vi "5668 Initialize Scan with External LO.vi"(8 "error in (no error)":errorcluster, 10 "Start Carrier Frequency (Hz)":dbl=4000000000.0 format="%#_13p", 11 "Instrument Handles in":T1={"Resource Name RFSA"="RFSA", "Resource Name RFSG LO Generation"="RFSG"}) -> (0 "error out":errorcluster, 3 "Instrument Handles out":T1={"Resource Name RFSA"="RFSA", "Resource Name RFSG LO Generation"="RFSG"})   [LabVIEW 2017]
uses:
  Instrument Handles.ctl
  <instrlib>/niRFSA/niRFSA.llb/niRFSA Acquisition Types.ctl
  <instrlib>/niRFSA/niRFSA.llb/niRFSA Ref Clock Sources.ctl
panel:
  in  "resource name":refnum<k15>="PXI1Slot17"
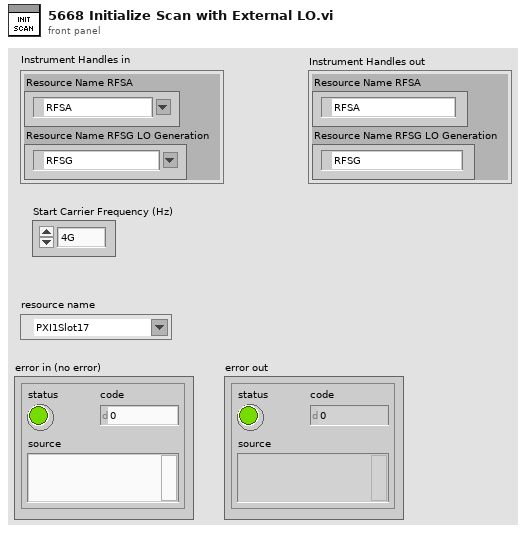
[diagram p1: front panel]
types:
  T1 = typedef "Instrument Handles.ctl" = cluster{"Resource Name RFSA":refnum<k15>, "Resource Name RFSG LO Generation":refnum<k15>}
  T2 = typedef "niRFSA Ref Clock Sources.ctl" = string
  T3 = typedef "niRFSA Acquisition Types.ctl" = i32
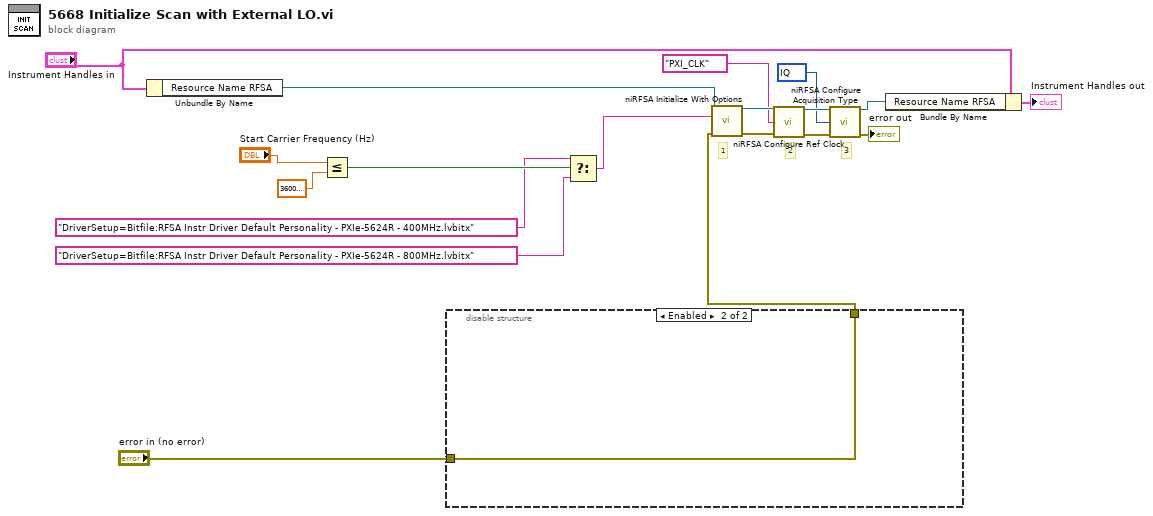
[diagram p0: block diagram]
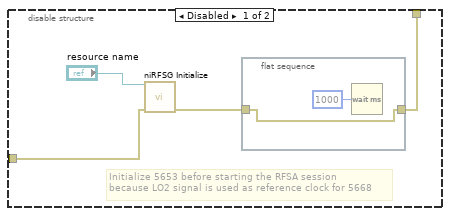
[diagram p2: hidden frame]
diagram:
  w14 = T3 100 items=["IQ"=100, "Spectrum"=101] ("acquisition type")
  # "3"
  # "2"
  # "1"
  n1 = Unbundle By Name("Instrument Handles in") -> ("Resource Name RFSA"=w12:refnum<k15>)
  n2 = Less Or Equal?(x="Start Carrier Frequency (Hz)", y=3600000000.0) -> (x <= y?=w10:bool)
  n3 = disable-structure shown="Enabled" {
    disable-tunnel: "error in (no error)" -> [w22 w26]
    disable-tunnel: [w20 w26] -> w1
    frame Disabled {
      # "Initialize 5653 before starting the RFSA session\nbecause LO2 signal is used as reference clock for 5668"
      n4 = call <instrlib>:"niRFSG Initialize.vi"("resource name"="resource name", "error in"=w22) -> ("error out"=w21:errorcluster)  [unwired: 12 in, 1 out]
      n5 = flat-sequence {
        tunnel: w21 -> [w24]
        tunnel: [w24] -> w20
        frame #0 {
          n6 = Wait (ms)(milliseconds to wait=u32 1000) -> ()  [unwired: 1 out]
        }
      }
    }
    frame Enabled {
    }
  }
  n7 = Select(t="DriverSetup=Bitfile:RFSA Instr Driver Default Personality - PXIe-5624R - 400MHz.lvbitx" ("option string"), s=w10, f="DriverSetup=Bitfile:RFSA Instr Driver Default Personality - PXIe-5624R - 800MHz.lvbitx" ("option string")) -> (s? t:f=w7:string)
  n8 = call <instrlib>:"niRFSA Initialize With Options.vi"("resource name"=w12, "option string"=w7, "error in"=w1) -> ("instrument handle out"=w19:refnum<k15>, "error out"=w18:errorcluster)  [unwired: 11 in]
  n9 = call <instrlib>:"niRFSA Configure Ref Clock.vi"("instrument handle"=w19, "clock source"=T2 "PXI_CLK" ("Clock Source"), "error in"=w18) -> ("instrument handle out"=w15:refnum<k15>, "error out"=w16:errorcluster)  [unwired: 11 in]
  n10 = call <instrlib>:"niRFSA Configure Acquisition Type.vi"("instrument handle"=w15, "acquisition type"=w14, "error in"=w16) -> ("instrument handle out"=w6:refnum<k15>, "error out"=→"error out":errorcluster)  [unwired: 11 in]
  n11 = Bundle By Name(cluster="Instrument Handles in", "Resource Name RFSA"=w6) -> (→"Instrument Handles out":T1)
